vi "Tailor Sequence.vi"(7 "Time Thre (1 ns)":dbl=1e-09 format="%#_6p", 9 "Tailor Empty End (TRUE)":bool=TRUE, 10 "Tailor Empty Start (TRUE)":bool=TRUE, 11 "8Channel Sequence in":T3(array[cluster])) -> (3 "8Channel Sequence out":T3(array[cluster]))   [LabVIEW 2020]
uses:
  Labview Library/Libraries/HW_LMMR_ASG8100/LMMR ASG/Loop Config.ctl
  Labview Library/Libraries/HW_LMMR_ASG8100/LMMR ASG/Loop Code.ctl
  Labview Library/Libraries/HW_LMMR_ASG8100/LMMR ASG/Loop XControl.xctl
panel:
  out "Abandon Array":T3(array[cluster])
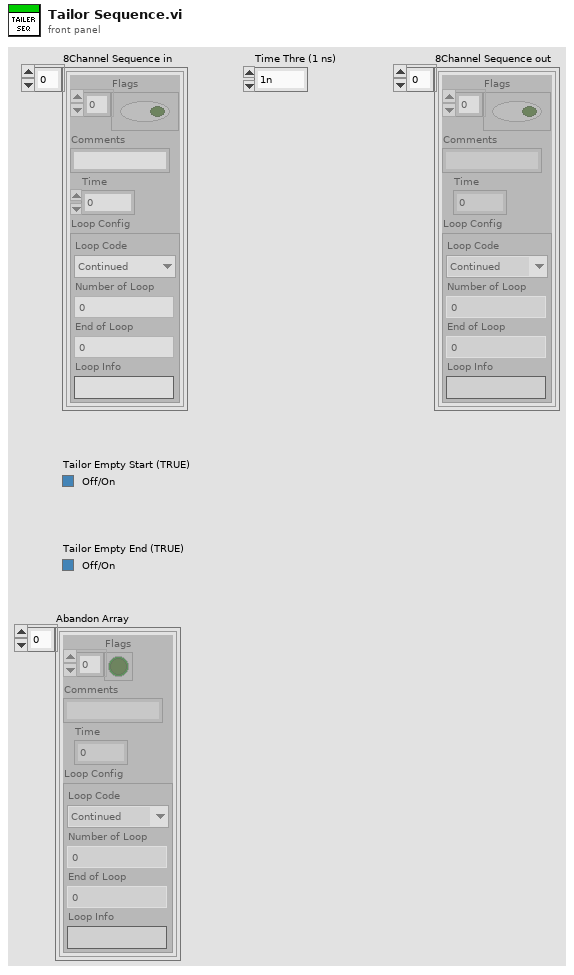
[diagram p1: front panel]
types:
  T1 = typedef "Loop XControl.xctl/Loop Config.ctl" = cluster{"Loop Code":T2, "Number of Loop":i32, "End of Loop":dbl, "Loop Info":string}
  T2 = typedef "Loop XControl.xctl/Loop Code.ctl" = enum16{"Continued", "Loop", "End Loop"}
  T3 = cluster{"Flags":bool[], "Comments":string, "Time":dbl, "Loop Config":T1}[]
  T4 = cluster{"Flags":bool[], "Comments":string, "Time":dbl, "Loop Config":T1}
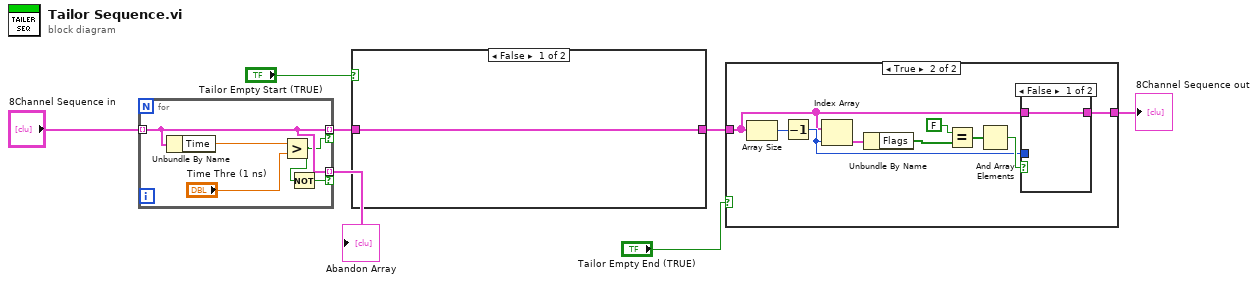
[diagram p0: block diagram]
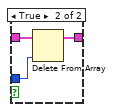
[diagram p3: hidden frame]
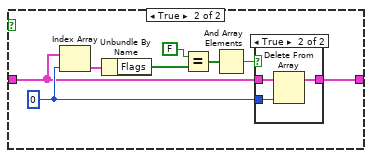
[diagram p4: hidden frame]
diagram:
  n1 = for {
    tunnel: "8Channel Sequence in" -> [w10] mode=indexing
    tunnel: [w10] -> w4 mode=indexing if=w8
    tunnel: [w10] -> w1 mode=indexing if=w9
    n2 = Unbundle By Name(w10) -> ("Time"=w12:dbl)
    n3 = Greater?(x=w12, y="Time Thre (1 ns)") -> (0:w8:bool)
    n4 = Not(x=w8) -> (.not. x?=w9:bool)
  }
  "Abandon Array" <- w1
  n5 = case shown="False" "Tailor Empty Start (TRUE)" {
    tunnel: [w13 w20] -> w6
    tunnel: w4 -> [w13 w14]
    frame False {
    }
    frame True {
      w19 = 0 ("index")
      n6 = Index Array(array=w14, index=w19) -> (element=w15:T4)
      n7 = Unbundle By Name(w15) -> ("Flags"=w16:bool[])
      n8 = Equal?(x=FALSE, y=w16) -> (x = y?=w18:bool[])
      n9 = And Array Elements(Boolean array=w18) -> (logical AND=w21:bool)
      n10 = case shown="True" w21 {
        tunnel: w19 -> [_ w25]
        tunnel: w14 -> [w22 w24]
        tunnel: [w22 w23] -> w20
        frame False {
        }
        frame True {
          n11 = Delete From Array(array=w24, index=w25) -> (array with subset deleted=w23:T3)  [unwired: 1 in, 1 out]
        }
      }
    }
  }
  n12 = case shown="True" "Tailor Empty End (TRUE)" {
    tunnel: [w26 w34] -> w7
    tunnel: w6 -> [w26 w31]
    frame False {
    }
    frame True {
      n13 = Array Size(array=w31) -> (size(s)=w32:i32)
      n14 = Decrement(x=w32) -> (x-1=w33:i32)
      n15 = Index Array(array=w31, index=w33) -> (element=w30:T4)
      n16 = Unbundle By Name(w30) -> ("Flags"=w29:bool[])
      n17 = Equal?(x=FALSE, y=w29) -> (x = y?=w27:bool[])
      n18 = And Array Elements(Boolean array=w27) -> (logical AND=w35:bool)
      n19 = case shown="False" w35 {
        tunnel: w31 -> [w36 w39]
        tunnel: w33 -> [_ w38]
        tunnel: [w36 w37] -> w34
        frame False {
        }
        frame True {
          n20 = Delete From Array(array=w39, index=w38) -> (array with subset deleted=w37:T3)  [unwired: 1 in, 1 out]
        }
      }
    }
  }
  "8Channel Sequence out" <- w7
